vi "Row-Swap 2D num Array.vi"(8 "Index b":i32=1, 9 "Index a":i32=1, 11 "row-swapped array":dbl[][](array[numeric])) -> (3 "row-swapped array":dbl[][](array[numeric]))   [LabVIEW 2010]
doc: "Swaps the rows of \"row-swapped array\" specified by Index a and Index b"
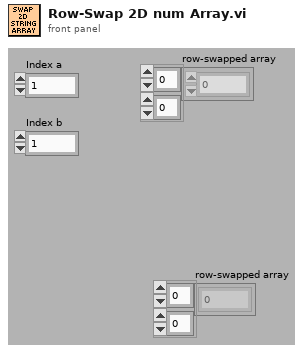
[diagram p1: front panel]
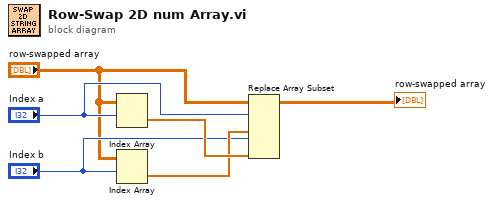
[diagram p0: block diagram]
diagram:
  n1 = Index Array(array="row-swapped array", index (row)="Index a") -> (element=w6:dbl[])  [unwired: 1 in]
  n2 = Index Array(array="row-swapped array", index (row)="Index b") -> (element=w5:dbl[])  [unwired: 1 in]
  n3 = Replace Array Subset "Replace Array Subset"(array="row-swapped array", new element #1=w5, index (row) #1="Index a", new element #2=w6, index (row) #2="Index b") -> (→"row-swapped array":dbl[][])  [unwired: 2 in]
